vi "BRig_RT__Case_Exp__State_endTrial.vi"(9 "input_timeStamp_start":dbl, 10 "input_dataTrial":u16[][](array[numeric]), 11 "input_dataCurrent":u16[](array[numeric])) -> (2 "output_dataTrial":u16[][](array[numeric]), 3 "output_dataCurrent":u16[](array[numeric]), 5 "output_runTime":dbl)   [LabVIEW 2014]
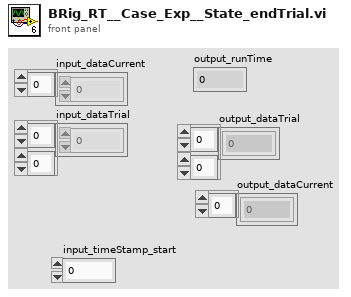
[diagram p1: front panel]
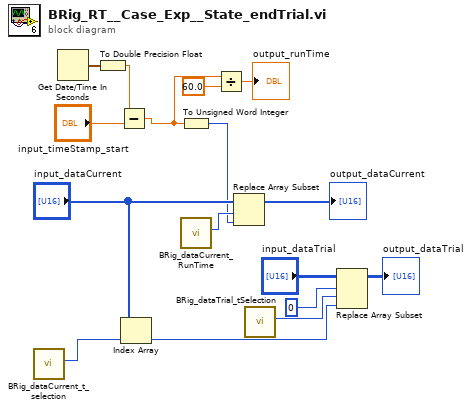
[diagram p0: block diagram]
diagram:
  n1 = call "BRig_dataCurrent_t_selection.vi"() -> ("output_t_selection"=w5:i32)  [unwired: 11 in]
  n2 = Get Date/Time In Seconds() -> (seconds since 1Jan1904=w11:timestamp)
  n3 = To Double Precision Float(number=w11) -> (double precision float=w9:dbl)
  n4 = Subtract(x=w9, y="input_timeStamp_start") -> (x-y=w3:dbl)
  n5 = Index Array(array="input_dataCurrent", index=w5) -> (element=w4:u16)
  n6 = To Unsigned Word Integer(number=w3) -> (unsigned 16bit integer=w8:u16)
  n7 = call "BRig_dataCurrent_RunTime.vi"() -> ("output_RunTime"=w12:i32)  [unwired: 11 in]
  n8 = Divide(x=w3, y=60.0) -> (x/y=→"output_runTime":dbl)
  n9 = Replace Array Subset(array="input_dataCurrent", new element=w8, index=w12) -> (→"output_dataCurrent":u16[])
  n10 = call "BRig_dataTrial_tSelection.vi"() -> ("output_tSelection"=w16:i32)  [unwired: 11 in]
  n11 = Replace Array Subset(array="input_dataTrial", new element=w4, index (row)=0, index (col)=w16) -> (→"output_dataTrial":u16[][])
